vi "luaL_loadstring.vi"(8 "error in (no error)":errorcluster, 10 "lua chunk":string="--Lua Script", 11 "lua_state_p":u64) -> (0 "error out":errorcluster, 3 "lua_state_p out":u64)   [LabVIEW 2020, in "lua.dll.lvlib"]
doc: "luaL_loadstring\n[-0, +1, –]\nint luaL_loadstring (lua_State *L, const char *s);\nLoads a string as a Lua chunk. This function uses lua_load to load the chunk in the zero-terminated string s.\n\nThis function returns the same results as lua_load.\n\nAlso as lua_load, this function only loads the chunk; it does not run it."
uses:
  lua.dll.lvlib
  lua_tolstring.vi
  lua54.dll
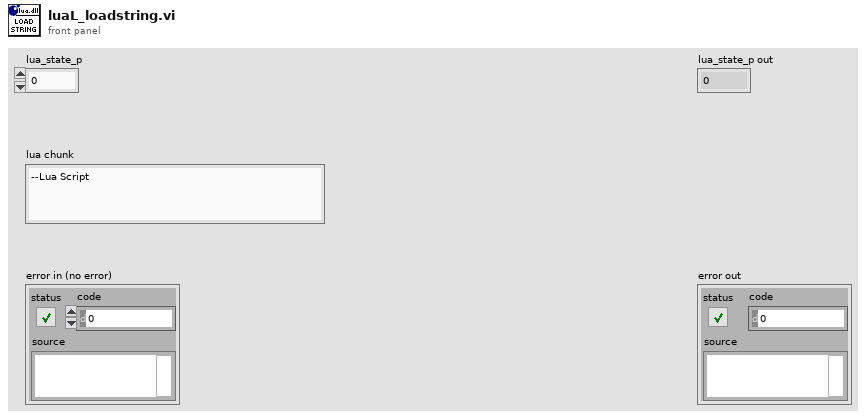
[diagram p1: front panel]
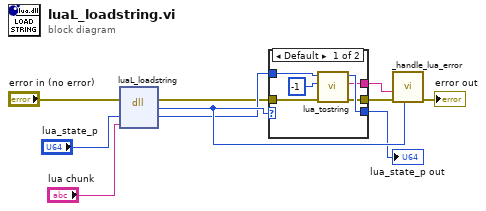
[diagram p0: block diagram]
diagram:
  n1 = dll-call lib="C:/Users/Nicholas Folse/Documents/workspace/github-tauterra.llc/Lua for LabVIEW/lib/lua.dll/lua54**.*" fn="luaL_loadstring"(error in="error in (no error)", "lua_state_p"="lua_state_p", "lua chunk"="lua chunk") -> (error out=w3:errorcluster, "errcode"=w6:i32, "lua_state_p"=w4:u64)  [unwired: 3 in, 1 out]
  n2 = case shown="Default" w6 {
    tunnel: [w15 w18] -> w5
    tunnel: w4 -> [w16 w18]
    tunnel: w3 -> [w14 w17]
    tunnel: [w13 w17] -> w2
    tunnel: [w11 _] -> w1
    frame Default {
      n3 = call "lua_tostring.vi"("error in (no error)"=w14, "index"=-1, "lua_state_p"=w16) -> ("error out"=w13:errorcluster, "string"=w11:string, "lua_state_p out"=w15:u64)  [unwired: 6 in]
    }
    frame 0 {
    }
  }
  "lua_state_p out" <- w5
  n4 = call "_handle_lua_error.vi"("lua status"=w6, "error in (no error)"=w2, "error string"=w1) -> ("error out"=→"error out":errorcluster)  [unwired: 8 in]
